vi "Measurement UI.vi"() -> ()   [LabVIEW 2022 SP3, in "Crosstalk Sweep_UI.lvlib"]
uses:
  Crosstalk Sweep_UI.lvlib
  shared/ui/controls/view.ctl
  shared/controls/digital output level units.ctl
  shared/controls/sweep profile.ctl
  UI State.ctl
  <vilib>/Utility/miscctls.llb/LVBoundsTypeDef.ctl
  <vilib>/Utility/miscctls.llb/LVPoint32TypeDef.ctl
  <vilib>/Utility/miscctls.llb/LVPointTypeDef.ctl
  shared/ui/UI Helpers.lvlib
  shared/audio popup ui/Audio Popup UI.lvlib
  shared/controls/audio controls.lvlib
panel:
  in  "view legend":T1
  out "plot point":string
  out "Sweep graph":cluster{"frequency (Hz)":dbl[], "THD+N":dbl[]}[](graph)
  out "Time domain graph":waveform(dbl)[](graph)
  out "Frequency domain graph":cluster{"f0":dbl, "df":dbl, "data":dbl[]}[](graph)
  in  "acq channel - interferrer":string="PXI1Slot4/ai0"
  in  "acq channel - victim":string="PXI1Slot4/ai1, PXI1Slot2/ai0:1"
  out "channel names":string[](array[string])
  in  "digital serial cfg file":string
  out "crosstalk (dB)":dbl[](array[numeric])
  out "frequency (Hz)":dbl[](array[numeric])
  in  "Configuration tab":enum32{"Protocol", "Measurement"}(tab)
  out "digital serial file name":string
  in  "configure digital serial":bool
  in  "master clock channel list":string caption="Master Clock Channel"
  in  "digital channel list":string caption="Digital Audio Channel"
  in  "sweep profile":T2=enum."Logarithmic" caption="Profile"
  in  "output level":dbl=-1.0 caption="Output level" format="%#_3f"
  in  "output level units":T3=enum."dBFS"
  in  "digital audio interferrer channel":i32 caption="Interferrer channel"
  in  "Interferrer channel resource":tag
  in  "Victim channel resource":tag
  in  "min settling cycles":u32 caption="Minimum settling cycles"
  in  "min settling time (s)":dbl=0.1 caption="Minimum settling time" format="%#_6ps"
  in  "number of steps":u32=20000 caption="Number of steps"
  in  "sweep start frequency (Hz)":dbl=20.0 caption="Sweep start" format="%#_6pHz"
  in  "sweep stop frequency (Hz)":dbl=20000.0 caption="Sweep stop" format="%#_6pHz"
  in  "min measurement cycles":u32 caption="Minimum measurement cycles"
  in  "acq sampling rate":dbl=51200.0 caption="Sample rate" format="%#.6pHz"
  in  "min measurement time (s)":dbl=0.1 caption="Minimum measurement time" format="%#_6ps"
  in  "lowpass filter":T4(ring) caption="Lowpass filter"
  in  "highpass filter":enum32{"DC", "AC"}(ring) caption="Highpass filter"
  in  "weighting filter":T5(ring)=enum."A-weighting" caption="Weighting filter"
  in  "load impedance":dbl=4.0 caption="Load impedance" format="%#_6p Ohms"
  in  "output range (pk-pk)":dbl=15.0 caption="Output range" format="%.3p Vpk-pk"
  out "fft - data":dbl[](array[numeric])
  out "fft - df":dbl
  out "fft - f0":dbl
  out "wfm - data":dbl[](array[numeric])
  out "wfm - dt":dbl
  out "wfm - t0":dbl
  in  "acq channel":string="PXI1Slot4/ai0"
  in  "signal phase":dbl caption="phase"
  # "hidden controls - used to sync with MeasLink"
  # "hidden indicators"
  # "Digital Serial Settings"
  # "Harware Resource"
  # "Filters"
  # "Output Sweep"
  # "Acquisition"
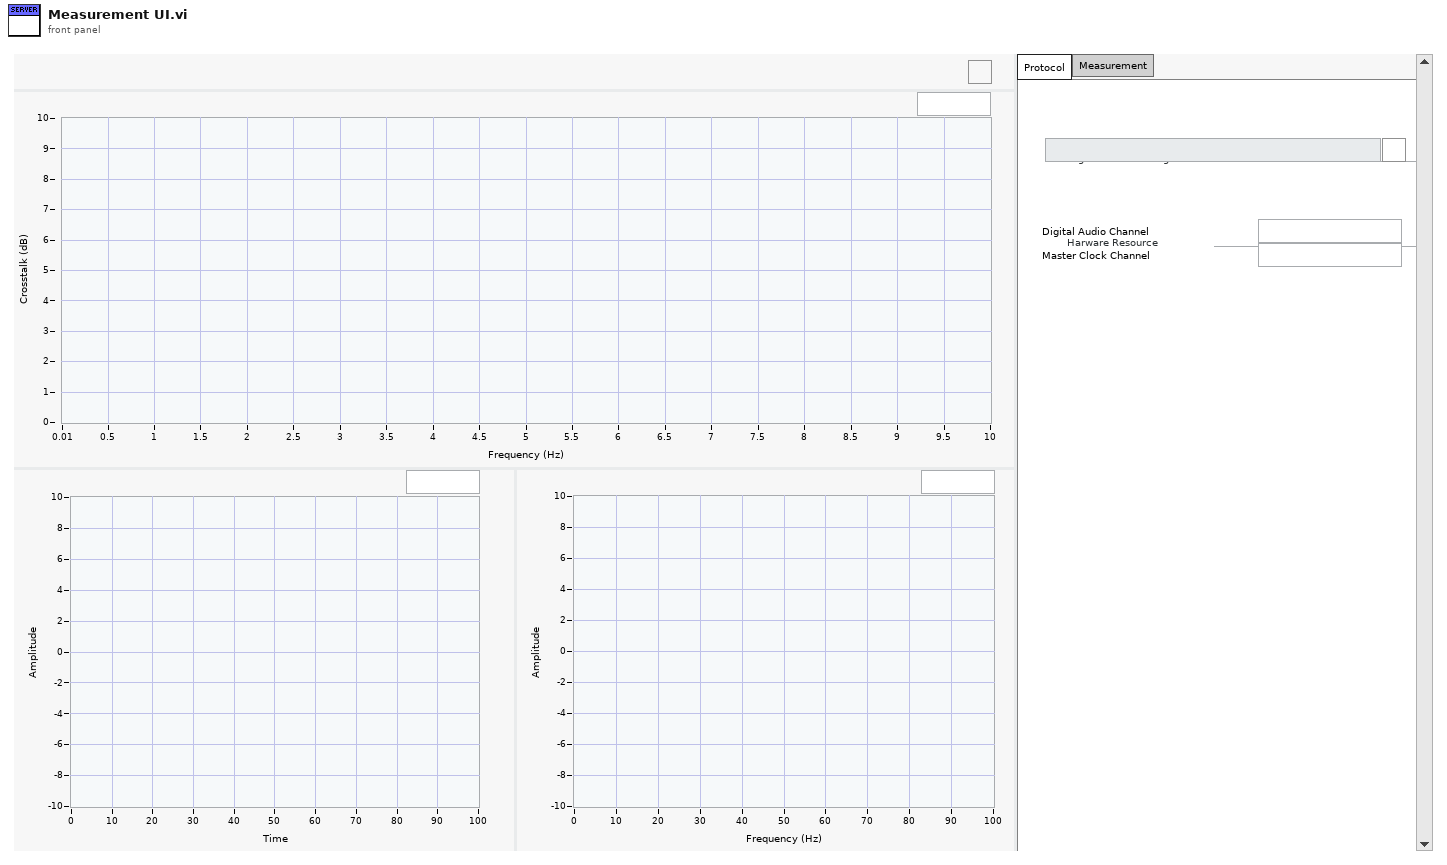
[diagram p1: front panel]
types:
  T1 = typedef "UI Helpers.lvlib/view.ctl" = bool
  T2 = typedef "audio controls.lvlib/sweep profile.ctl" = enum32{"Linear", "Logarithmic"}
  T3 = typedef "audio controls.lvlib/digital output level units.ctl" = enum32{"% FS", "dBFS", "V"}
  T4 = enum32{"No filter", "AES17 20kHz", "AES17 40kHz"}
  T5 = enum32{"Linear", "A-weighting", "B-weighting", "C-weighting"}
  T6 = typedef "Crosstalk Sweep_UI.lvlib/UI State.ctl" = cluster{"Graph Size":T7, "Legend Visible":bool, "Mouse Coords":T8, "Visible Plot Id":i32, "PostUI event occurred":bool, "digital serial cfg file":path}
  T7 = typedef "LVBoundsTypeDef.ctl" = cluster{"Width":u32, "Height":u32}
  T8 = typedef "LVPoint32TypeDef.ctl" = cluster{"Horizontal":i32, "Vertical":i32}
  T9 = typedef "LVPointTypeDef.ctl" = cluster{"Horizontal":i16, "Vertical":i16}
  T10 = typedef "Audio Popup UI.lvlib/audio settings.ctl" = cluster{"digital serial file":string}
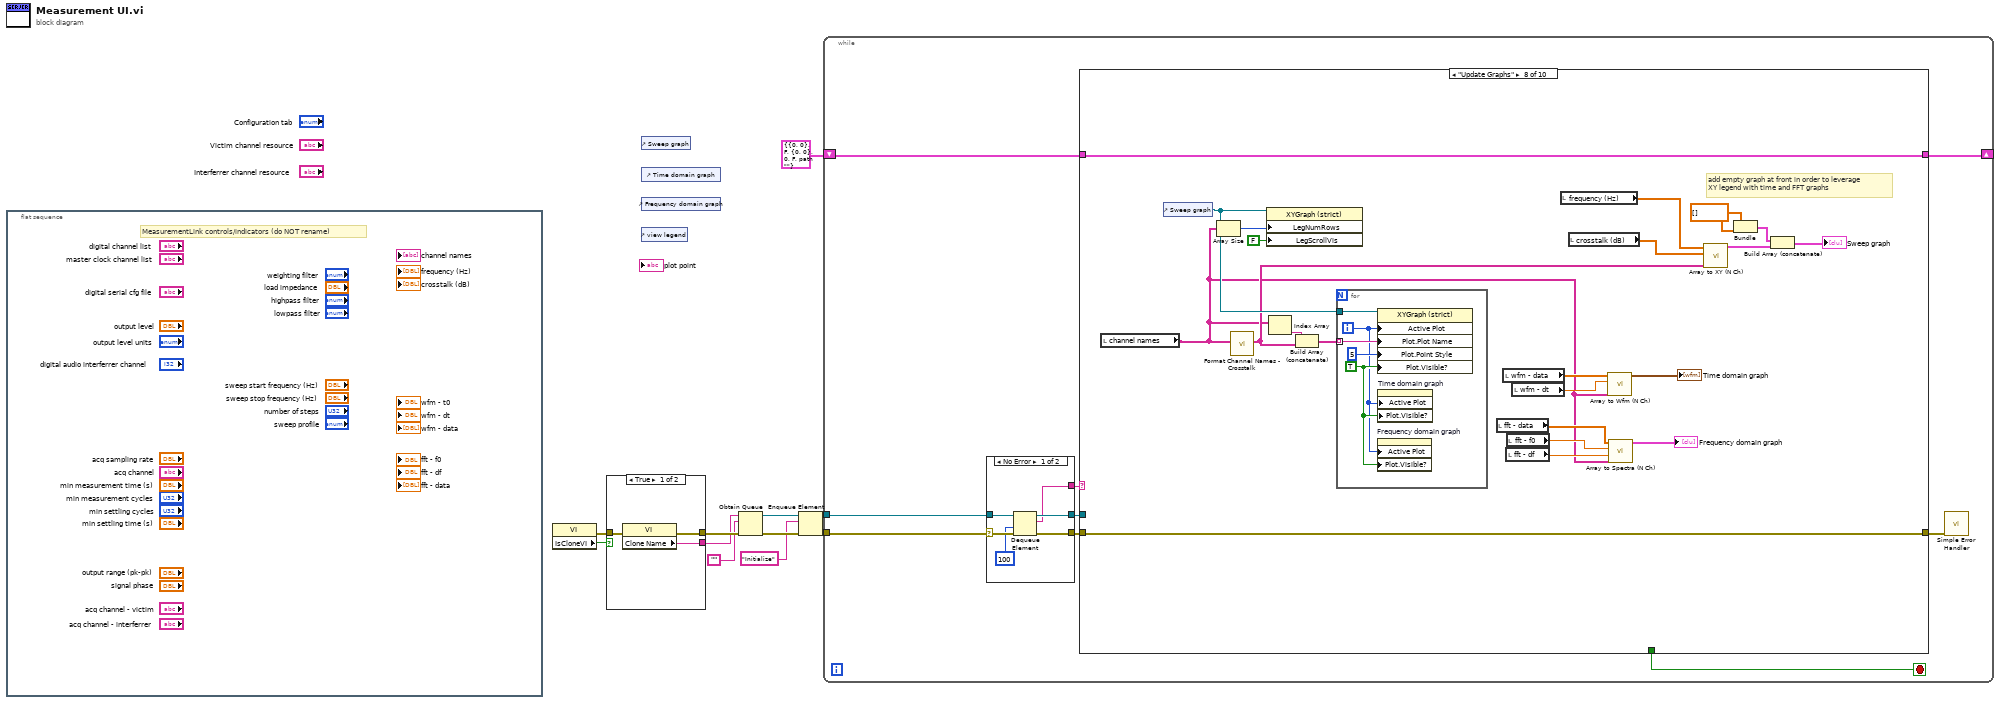
[diagram p0: block diagram]
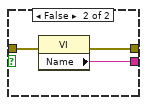
[diagram p2: hidden frame]
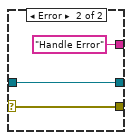
[diagram p3: hidden frame]
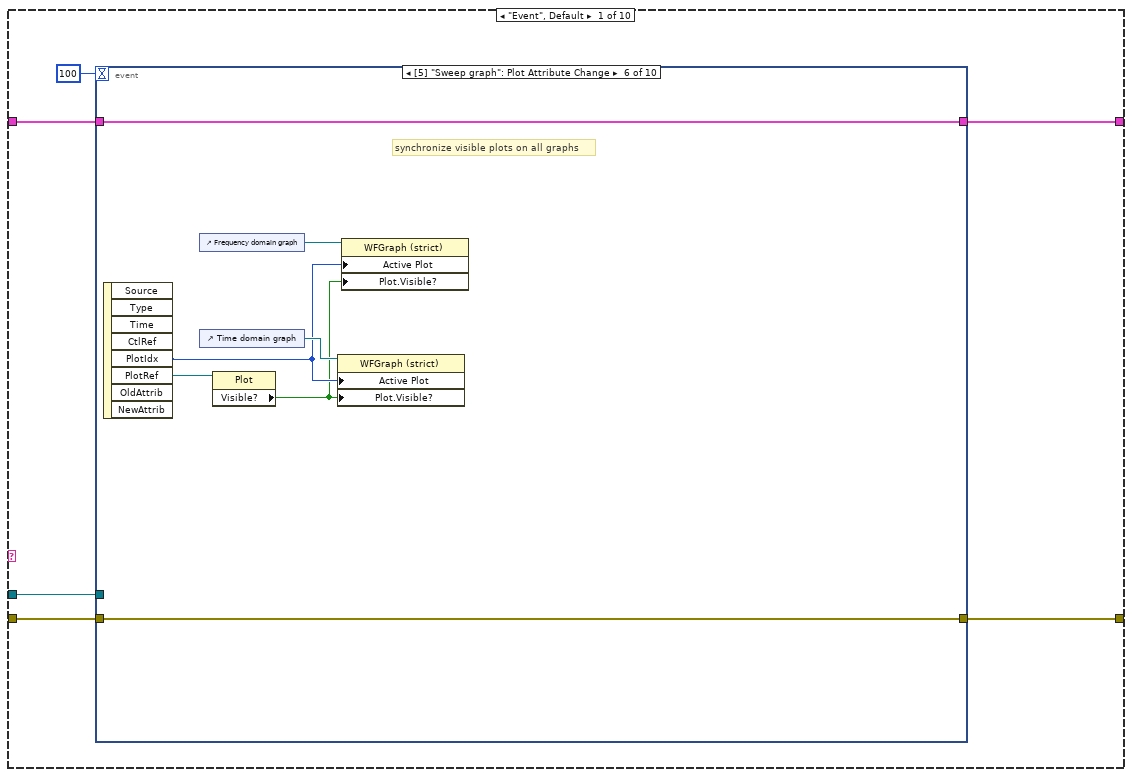
[diagram p4: hidden frame]
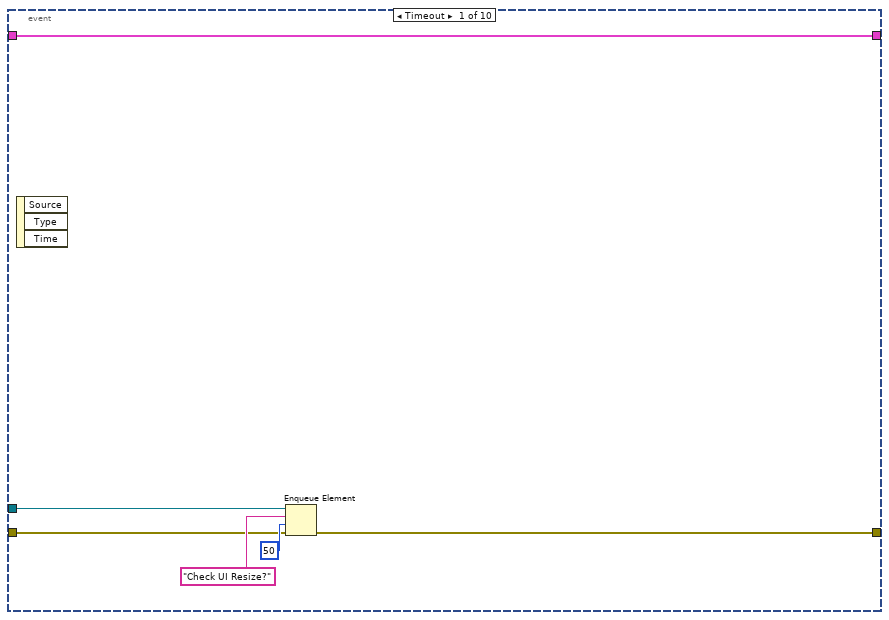
[diagram p5: hidden frame]
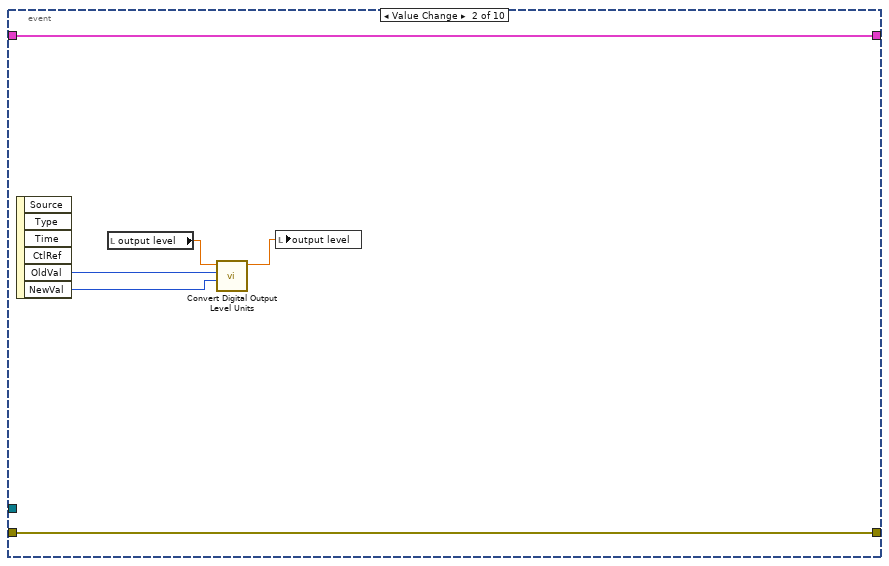
[diagram p6: hidden frame]
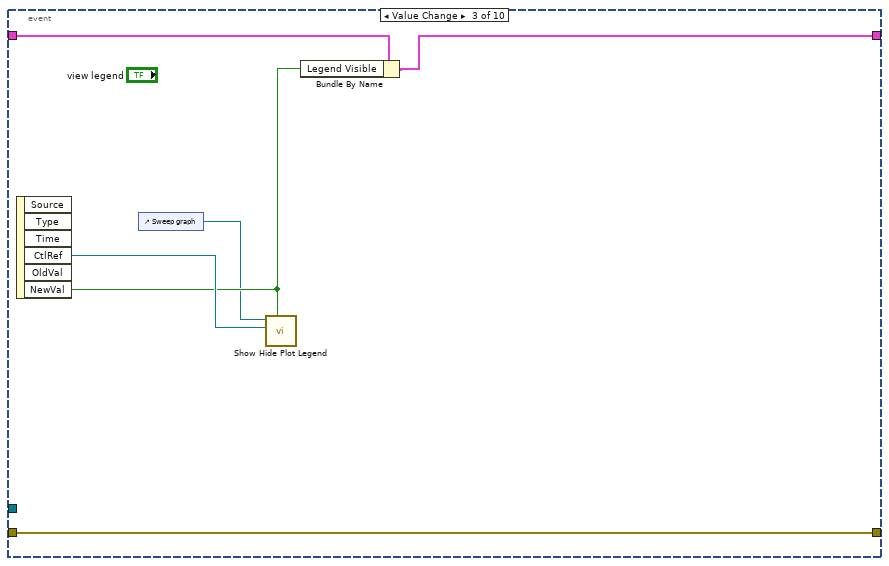
[diagram p7: hidden frame]
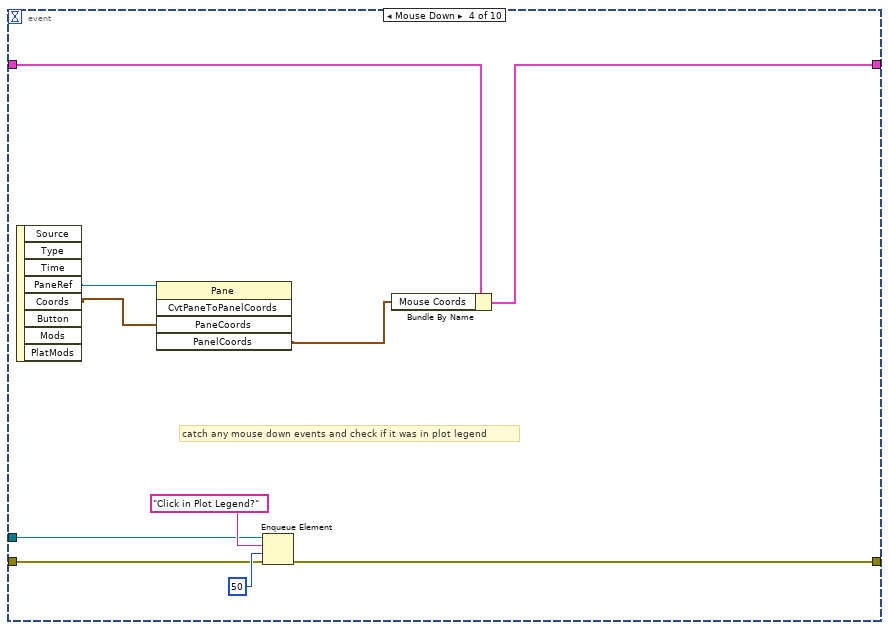
[diagram p8: hidden frame]
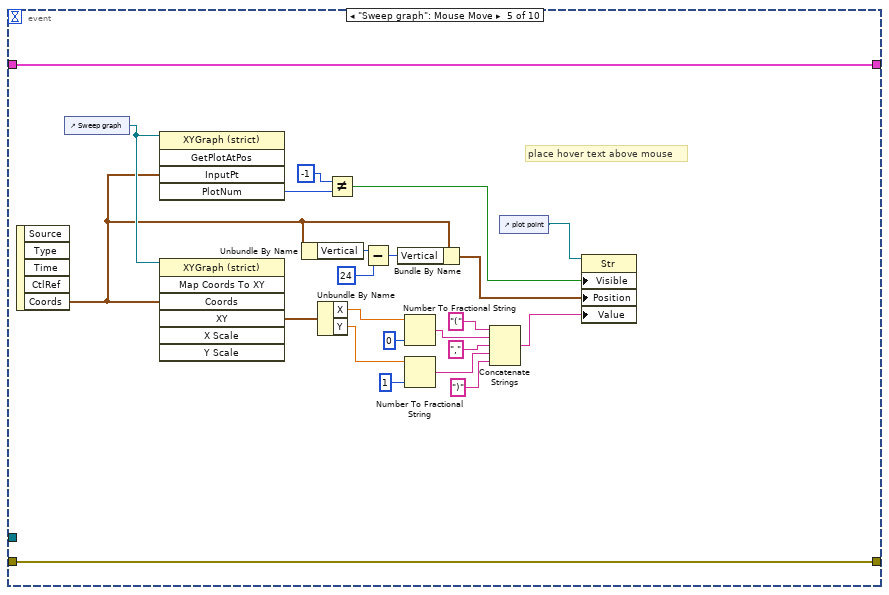
[diagram p9: hidden frame]
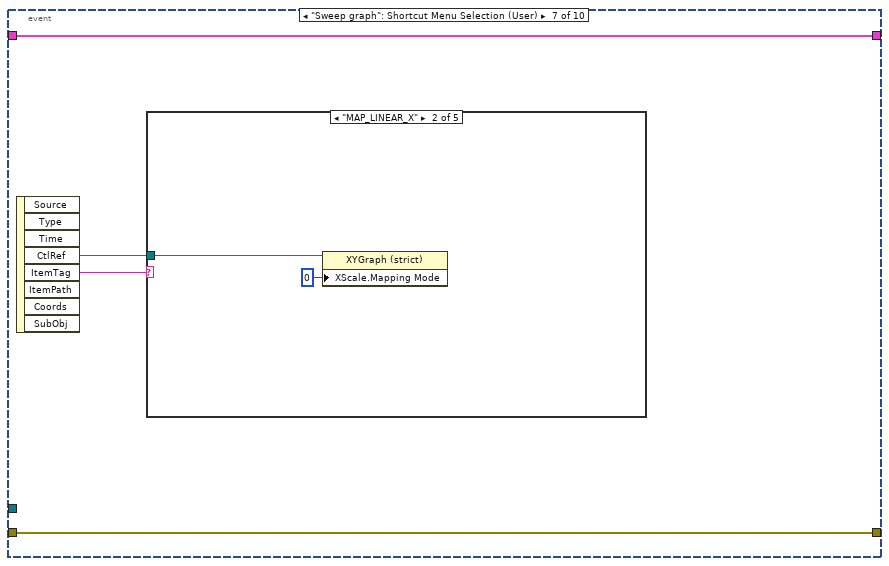
[diagram p10: hidden frame]
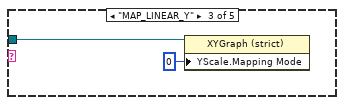
[diagram p12: hidden frame]
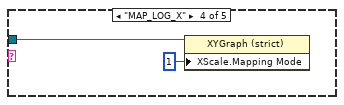
[diagram p13: hidden frame]
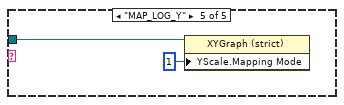
[diagram p14: hidden frame]
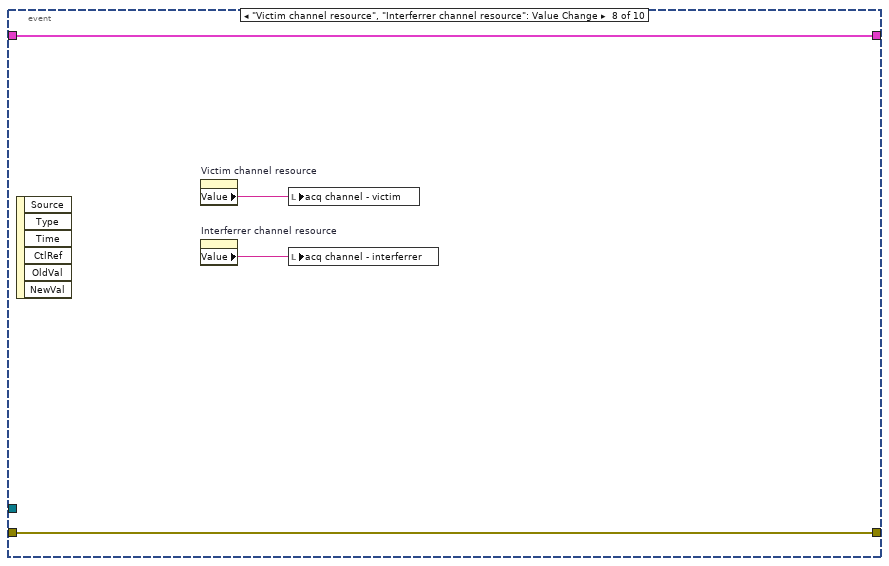
[diagram p15: hidden frame]
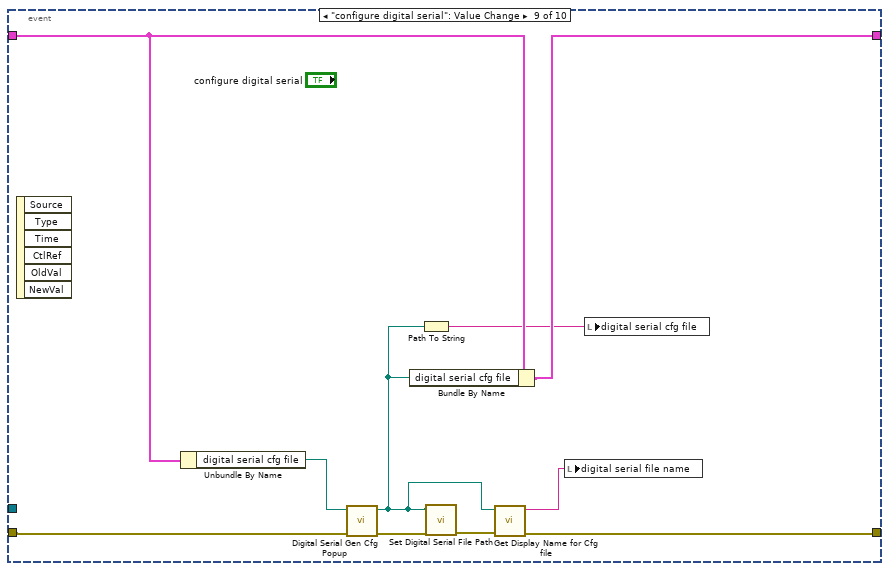
[diagram p16: hidden frame]
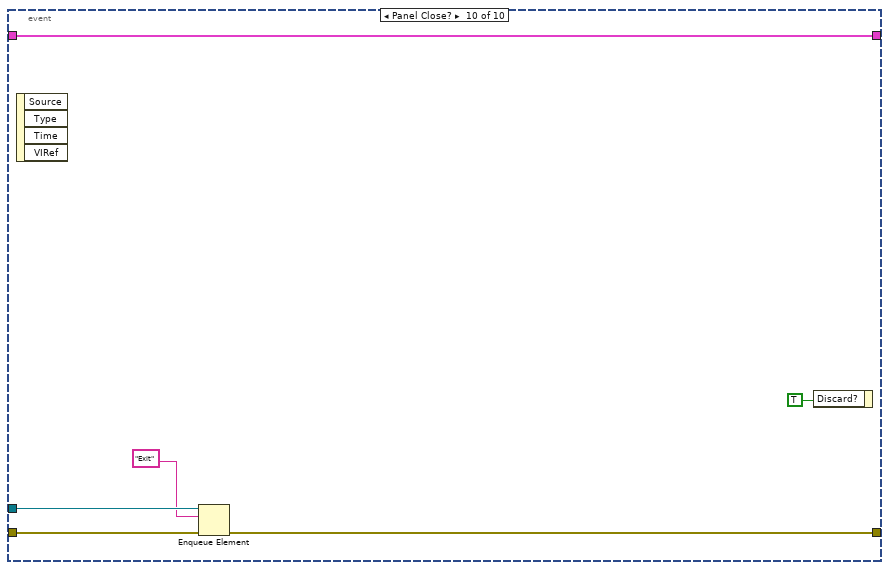
[diagram p17: hidden frame]
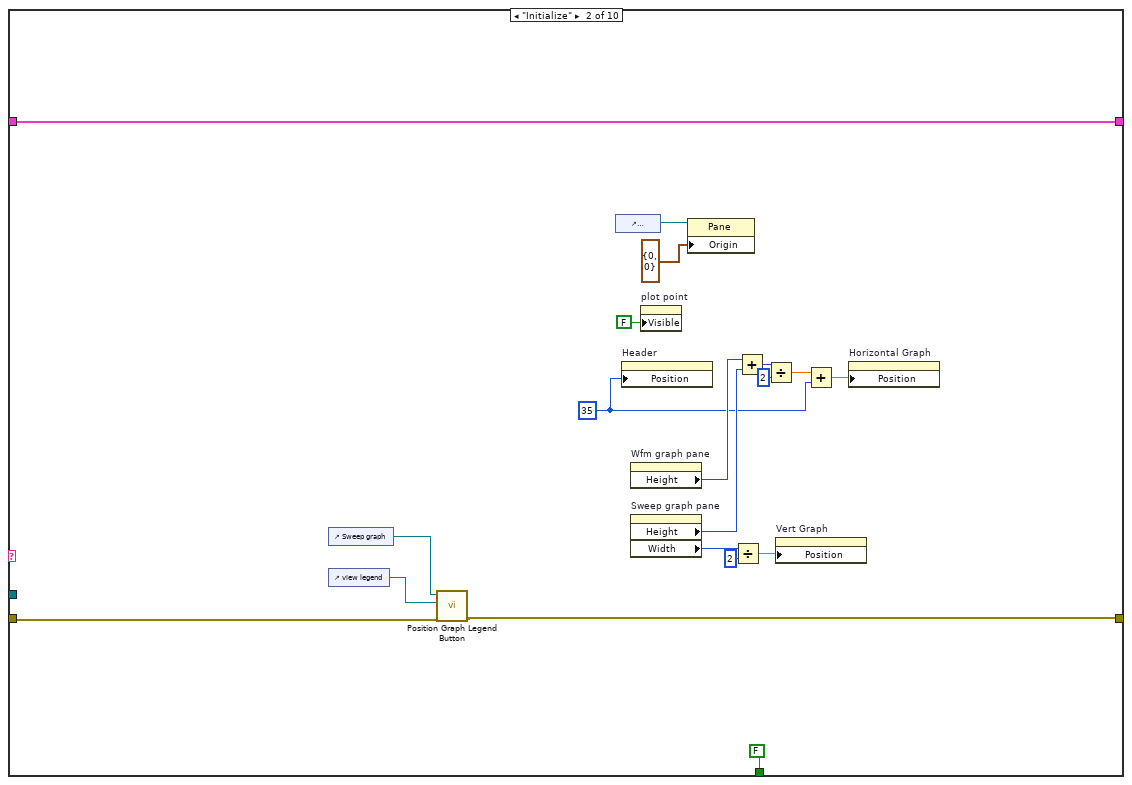
[diagram p18: hidden frame]
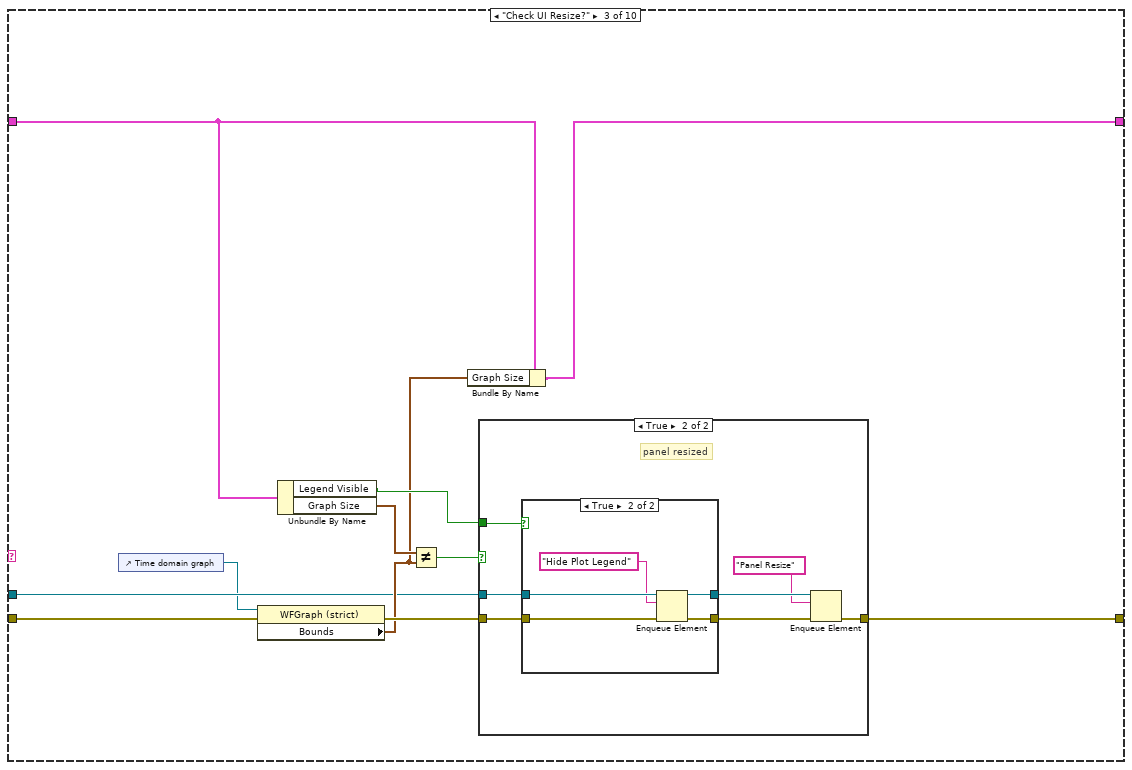
[diagram p19: hidden frame]
diagram:
  n1 = flat-sequence {
    frame #0 {
      # "MeasurementLink controls/indicators (do NOT rename)"
    }
  }
  n2 = property class="VI"() -> (error out=w2:errorcluster, "IsCloneVI"=w3:bool)  [unwired: 2 in, 1 out]
  n3 = case shown="True" w3 {
    tunnel: [w14 w17] -> w11
    tunnel: [w13 w16] -> w10
    tunnel: w2 -> [w12 w15]
    frame True {
      n4 = property class="VI"(error in=w12) -> (error out=w14:errorcluster, "Clone Name"=w13:string)  [unwired: 1 in, 1 out]
    }
    frame False {
      n5 = property class="VI"(error in=w15) -> (error out=w17:errorcluster, "Name"=w16:string)  [unwired: 1 in, 1 out]
    }
  }
  n6 = control-ref of="Sweep graph"() -> ()  [unwired: 1 out]
  n7 = control-ref of="Time domain graph"() -> ()  [unwired: 1 out]
  n8 = control-ref of="Frequency domain graph"() -> ()  [unwired: 1 out]
  n9 = control-ref of="view legend"() -> ()  [unwired: 1 out]
  n10 = Obtain Queue(name (unnamed)=w10, element data type="", error in (no error)=w11) -> (queue out=w7:refnum<queue>, error out=w9:errorcluster)  [unwired: 2 in, 1 out]
  n11 = Enqueue Element(queue=w7, element="Initialize", error in (no error)=w9) -> (queue out=w6:refnum<queue>, error out=w8:errorcluster)  [unwired: 1 in, 1 out]
  n12 = while {
    tunnel: w6 -> [w24]
    shift-right: [w20] -> _
    shift-left: T6 {"Graph Size"={"Width"=0, "Height"=0}, "Legend Visible"=FALSE, "Mouse Coords"={"Horizontal"=0, "Vertical"=0}, "Visible Plot Id"=0, "PostUI event occurred"=FALSE, "digital serial cfg file"=path ""} ("UI State") -> [w19]
    tunnel: w8 -> [w26]
    stop <- w21 stop-if-true
    n13 = case shown="No Error" w26 {
      selector: w26 -> [w32 w35]
      tunnel: [w31 w35] -> w25
      tunnel: w24 -> [w30 w34]
      tunnel: [w29 w34] -> w23
      tunnel: [w28 "Handle Error"] -> w22
      frame No Error {
        n14 = Dequeue Element(queue=w30, timeout in ms (-1)=100, error in (no error)=w32) -> (queue out=w29:refnum<queue>, element=w28:string, error out=w31:errorcluster)  [unwired: 1 out]
      }
      frame Error {
      }
    }
    n15 = case shown="\"Update Graphs\"" w22 {
      tunnel: w25 -> [w40 w133 w155 w179 w199 w207 w215 w251 w277 w279]
      tunnel: w23 -> [w38 _ w156 w180 _ _ w214 _ w275 _]
      tunnel: [w41 w132 w154 w178 w198 w204 w209 w251 w272 w279] -> w18
      tunnel: [_ FALSE _ _ _ _ _ _ TRUE _] -> w21
      tunnel: [w36 w134 w151 w177 w201 w208 w212 w264 w270 w278] -> w20
      tunnel: w19 -> [w37 w134 w152 w177 w202 w208 w213 w264 w270 w278]
      frame "Event", Default {
        n16 = event shown="[5] \"Sweep graph\": Plot Attribute Change" {
          selector: _ -> [_ _ _ _ _ _ _ _ _ _]
          dyn-events: _ -> [_ _ _ _ _ _ _ _ _ _]
          timeout: 100 -> [_ _ _ _ _ _ _ _ _ _]
          tunnel: [w44 w53 w59 w65 w92 w98 w103 w114 w116 w129] -> w41
          tunnel: w40 -> [w45 w53 w59 w67 w92 w98 w103 w114 w121 w130]
          tunnel: w38 -> [w43 _ _ w66 _ _ _ _ _ w128]
          tunnel: w37 -> [w42 w52 w56 w64 w91 w97 w102 w115 w120 w126]
          tunnel: [w42 w52 w55 w63 w91 w97 w102 w115 w119 w126] -> w36
          event Timeout {
            n17 = event-data() -> ()  [unwired: 1 in, 3 out]
            n18 = Enqueue Element(queue=w43, element="Check UI Resize?", timeout in ms (-1)=50, error in (no error)=w45) -> (error out=w44:errorcluster)  [unwired: 2 out]
          }
          event Value Change {
            n19 = event-data() -> ("OldVal"=w50:T3, "NewVal"=w49:T3)  [unwired: 1 in, 4 out]
            n20 = local read "output level"() -> (w51:dbl)
            n21 = call "Convert Digital Output Level Units.vi"("new output level units"=w49, "previous output level units"=w50, "previous output level"=w51) -> ("new output level"=w48:dbl)  [unwired: 8 in]
            n22 = local write "output level"(w48) -> ()
          }
          event Value Change {
            n23 = event-data() -> ("CtlRef"=w58:refnum<vi>, "NewVal"=w57:T1)  [unwired: 1 in, 4 out]
            n24 = control-ref of="Sweep graph"() -> (w54:refnum<vi>)
            n25 = call "Show Hide Plot Legend.vi"("show"=w57, "view reference"=w58, "graph reference"=w54) -> ()  [unwired: 8 in, 1 out]
            n26 = Bundle By Name(cluster=w56, "Legend Visible"=w57) -> (w55:T6)
          }
          event Mouse Down {
            # "catch any mouse down events and check if it was in plot legend"
            n27 = event-data() -> ("PaneRef"=w62:refnum<vi>, "Coords"=w61:T8)  [unwired: 1 in, 6 out]
            n28 = invoke class="Pane" method="CvtPaneToPanelCoords"(reference=w62, "PaneCoords"=w61) -> ("PanelCoords"=w60:T9)  [unwired: 3 in, 4 out]
            n29 = Enqueue Element(queue=w66, element="Click in Plot Legend?", timeout in ms (-1)=50, error in (no error)=w67) -> (error out=w65:errorcluster)  [unwired: 2 out]
            n30 = Bundle By Name(cluster=w64, "Mouse Coords"=w60) -> (w63:T6)
          }
          event "Sweep graph": Mouse Move {
            # "place hover text above mouse"
            n31 = event-data() -> ("Coords"=w71:T8)  [unwired: 1 in, 4 out]
            n32 = control-ref of="Sweep graph"() -> (w72:refnum<vi>)
            n33 = invoke class="XYGraph (strict)" method="GetPlotAtPos"(reference=w72, "InputPt"=w71) -> ("PlotNum"=w89:i32)  [unwired: 3 in, 4 out]
            n34 = invoke class="XYGraph (strict)" method="Map Coords To XY"(reference=w72, "Coords"=w71) -> ("XY"=w90:cluster{"X":dbl, "Y":dbl})  [unwired: 5 in, 6 out]
            n35 = Unbundle By Name(w71) -> ("Vertical"=w76:i32)
            n36 = Unbundle By Name(w90) -> ("X"=w79:dbl, "Y"=w78:dbl)
            n37 = Not Equal?(x=-1, y=w89) -> (x != y?=w87:bool)
            n38 = Subtract(x=w76, y=24) -> (x-y=w75:i32)
            n39 = Bundle By Name(cluster=w71, "Vertical"=w75) -> (w77:T8)
            n40 = Number To Fractional String(number=w79, precision (6)=i16 0) -> (F-format string=w85:string)  [unwired: 2 in]
            n41 = Number To Fractional String(number=w78, precision (6)=i16 1) -> (F-format string=w83:string)  [unwired: 2 in]
            n42 = Concatenate Strings("(" ("string"), w85, "," ("string"), w83, ")" ("string")) -> (w80:string)
            n43 = control-ref of="plot point"() -> (w73:refnum<vi>)
            n44 = property on="Property Node" class="Str"(reference=w73, "Visible"=w87, "Position"=w77, "Value"=w80) -> ()  [unwired: 1 in, 2 out]
          }
          event "Sweep graph": Plot Attribute Change {
            # "synchronize visible plots on all graphs"
            n45 = event-data() -> ("PlotIdx"=w94:i32, "PlotRef"=w99:refnum<vi>)  [unwired: 1 in, 6 out]
            n46 = control-ref of="Frequency domain graph"() -> (w95:refnum<vi>)
            n47 = control-ref of="Time domain graph"() -> (w96:refnum<vi>)
            n48 = property class="Plot"(reference=w99) -> ("Visible?"=w93:bool)  [unwired: 1 in, 2 out]
            n49 = property on="Property Node" class="WFGraph (strict)"(reference=w96, "Active Plot"=w94, "Plot.Visible?"=w93) -> ()  [unwired: 1 in, 2 out]
            n50 = property on="Property Node" class="WFGraph (strict)"(reference=w95, "Active Plot"=w94, "Plot.Visible?"=w93) -> ()  [unwired: 1 in, 2 out]
          }
          event "Sweep graph": Shortcut Menu Selection (User) {
            n51 = event-data() -> ("CtlRef"=w100:refnum<vi>, "ItemTag"=w101:string)  [unwired: 1 in, 6 out]
            n52 = case shown="\"MAP_LINEAR_X\"" w101 {
              tunnel: w100 -> [_ w105 w107 w109 w111]
              frame "", Default {
              }
              frame "MAP_LINEAR_X" {
                n53 = property class="XYGraph (strict)"(reference=w105, "XScale.Mapping Mode"=u8 0 ("X Scale.Mapping Mode")) -> ()  [unwired: 1 in, 2 out]
              }
              frame "MAP_LINEAR_Y" {
                n54 = property class="XYGraph (strict)"(reference=w107, "YScale.Mapping Mode"=u8 0 ("X Scale.Mapping Mode")) -> ()  [unwired: 1 in, 2 out]
              }
              frame "MAP_LOG_X" {
                n55 = property class="XYGraph (strict)"(reference=w109, "XScale.Mapping Mode"=u8 1 ("X Scale.Mapping Mode")) -> ()  [unwired: 1 in, 2 out]
              }
              frame "MAP_LOG_Y" {
                n56 = property class="XYGraph (strict)"(reference=w111, "YScale.Mapping Mode"=u8 1 ("X Scale.Mapping Mode")) -> ()  [unwired: 1 in, 2 out]
              }
            }
          }
          event "Victim channel resource", "Interferrer channel resource": Value Change {
            n57 = event-data() -> ()  [unwired: 1 in, 6 out]
            n58 = property on="Victim channel resource" class="DAQmxName"() -> ("Value"=w112:string)  [unwired: 2 in, 2 out]
            n59 = property on="Interferrer channel resource" class="DAQmxName"() -> ("Value"=w113:string)  [unwired: 2 in, 2 out]
            n60 = local write "acq channel - victim"(w112) -> ()
            n61 = local write "acq channel - interferrer"(w113) -> ()
          }
          event "configure digital serial": Value Change {
            n62 = event-data() -> ()  [unwired: 1 in, 6 out]
            n63 = Unbundle By Name(w120) -> ("digital serial cfg file"=w125:path)
            n64 = call "Digital Serial Gen Cfg Popup.vi"("error in (no error)"=w121, "config file in"=w125) -> ("error out"=w124:errorcluster, "config file out"=w122:path)  [unwired: 7 in, 1 out]
            n65 = Bundle By Name(cluster=w120, "digital serial cfg file"=w122) -> (w119:T6)
            n66 = Path To String(path=w122) -> (string=w118:string)
            n67 = call "Set Digital Serial File Path.vi"("error in (no error)"=w124, "digital serial file"=w122) -> ("error out"=w123:errorcluster)  [unwired: 9 in]
            n68 = call "Get Display Name for Cfg file.vi"("error in (no error)"=w123, "file path"=w122) -> ("error out"=w116:errorcluster, "display string"=w117:string)  [unwired: 8 in]
            n69 = local write "digital serial file name"(w117) -> ()
            n70 = local write "digital serial cfg file"(w118) -> ()
          }
          event Panel Close? {
            n71 = event-data() -> ()  [unwired: 1 in, 4 out]
            n72 = Enqueue Element(queue=w128, element="Exit", error in (no error)=w130) -> (error out=w129:errorcluster)  [unwired: 1 in, 2 out]
            n73 = event-data("Discard?"=TRUE) -> ()  [unwired: 1 in, 1 out]
          }
        }
      }
      frame "Initialize" {
        w138 = 35 ("Splitter Position")
        n74 = control-ref of="Sweep graph"() -> (w139:refnum<vi>)
        n75 = control-ref of="view legend"() -> (w149:refnum<vi>)
        n76 = call "Position Graph Legend Button.vi"("error in (no error)"=w133, "view legend"=w149, "graph"=w139) -> ("error out"=w132:errorcluster)  [unwired: 8 in]
        n77 = control-ref of="Configuration Pane"() -> (w137:refnum<vi>)
        n78 = property on="Header" class="Splitter"("Position"=w138) -> ()  [unwired: 2 in, 2 out]
        n79 = property on="Wfm graph pane" class="Pane"() -> ("Height"=w142:u32)  [unwired: 2 in, 2 out]
        n80 = property on="Sweep graph pane" class="Pane"() -> ("Height"=w141:u32, "Width"=w144:u32)  [unwired: 2 in, 2 out]
        n81 = property on="plot point" class="Str"("Visible"=FALSE) -> ()  [unwired: 2 in, 2 out]
        n82 = property class="Pane"(reference=w137, "Origin"=T9 {"Horizontal"=0, "Vertical"=0}) -> ()  [unwired: 1 in, 2 out]
        n83 = Divide(x=w144, y=2) -> (x/y=w143:dbl)
        n84 = Add(x=w142, y=w141) -> (x+y=w140:u32)
        n85 = Divide(x=w140, y=2) -> (x/y=w147:dbl)
        n86 = property on="Vert Graph" class="Splitter"("Position"=w143) -> ()  [unwired: 2 in, 2 out]
        n87 = Add(x=w147, y=w138) -> (x+y=w146:dbl)
        n88 = property on="Horizontal Graph" class="Splitter"("Position"=w146) -> ()  [unwired: 2 in, 2 out]
      }
      frame "Check UI Resize?" {
        n89 = control-ref of="Time domain graph"() -> (w153:refnum<vi>)
        n90 = property on="Property Node" class="WFGraph (strict)"(reference=w153, error in=w155) -> (error out=w161:errorcluster, "Bounds"=w157:T7)  [unwired: 1 out]
        n91 = Unbundle By Name(w152) -> ("Legend Visible"=w159:bool, "Graph Size"=w158:T7)
        n92 = Not Equal?(x=w158, y=w157) -> (x != y?=w160:bool)
        n93 = Bundle By Name(cluster=w152, "Graph Size"=w157) -> (w151:T6)
        n94 = case shown="True" w160 {
          tunnel: w161 -> [w162 w169]
          tunnel: [w162 w164] -> w154
          tunnel: w159 -> [_ w167]
          tunnel: w156 -> [_ w168]
          frame False {
            # "no resize"
          }
          frame True {
            # "panel resized"
            n95 = case shown="True" w167 {
              tunnel: w169 -> [w171 w176]
              tunnel: [w171 w175] -> w166
              tunnel: w168 -> [w170 w174]
              tunnel: [w170 w172] -> w165
              frame False {
              }
              frame True {
                n96 = Enqueue Element(queue=w174, element="Hide Plot Legend", error in (no error)=w176) -> (queue out=w172:refnum<queue>, error out=w175:errorcluster)  [unwired: 1 in, 1 out]
              }
            }
            n97 = Enqueue Element(queue=w165, element="Panel Resize", error in (no error)=w166) -> (error out=w164:errorcluster)  [unwired: 1 in, 2 out]
          }
        }
      }
      frame "Click in Plot Legend?" {
        n98 = Unbundle By Name(w177) -> ("Legend Visible"=w181:bool, "Mouse Coords"=w182:T8)
        n99 = case shown="True" w181 {
          tunnel: w182 -> [_ w189]
          tunnel: w180 -> [_ w186]
          tunnel: w179 -> [w183 w190]
          tunnel: [w183 w185] -> w178
          frame False {
            # "legend not visible; do nothing"
          }
          frame True {
            # "check if mouse down in legend"
            n100 = control-ref of="Sweep graph"() -> (w184:refnum<vi>)
            n101 = call "Check if Click in Graph Legend.vi"("error in (no error)"=w190, "Mouse Coords"=w189, "WaveformGraph"=w184) -> ("error out"=w187:errorcluster, "click in legend?"=w188:bool)  [unwired: 7 in]
            n102 = case shown="True" w188 {
              tunnel: w187 -> [w194 w195]
              tunnel: w186 -> [w193 _]
              tunnel: [w192 w195] -> w185
              frame False {
                n103 = Enqueue Element(queue=w193, element="Hide Plot Legend", error in (no error)=w194) -> (error out=w192:errorcluster)  [unwired: 1 in, 2 out]
              }
              frame True {
                # "inside legend; do nothing"
              }
            }
          }
        }
      }
      frame "Hide Plot Legend" {
        n104 = control-ref of="Sweep graph"() -> (w196:refnum<vi>)
        n105 = control-ref of="view legend"() -> (w197:refnum<vi>)
        n106 = call "Show Hide Plot Legend.vi"("show"=FALSE, "error in (no error)"=w199, "view reference"=w197, "graph reference"=w196) -> ("error out"=w198:errorcluster)  [unwired: 7 in]
        n107 = Bundle By Name(cluster=w202, "Legend Visible"=FALSE ("legend visible")) -> (w201:T6)
      }
      frame "Panel Resize" {
        n108 = control-ref of="Sweep graph"() -> (w206:refnum<vi>)
        n109 = control-ref of="view legend"() -> (w205:refnum<vi>)
        n110 = call "Position Graph Legend Button.vi"("error in (no error)"=w207, "view legend"=w205, "graph"=w206) -> ("error out"=w204:errorcluster)  [unwired: 8 in]
      }
      frame "Post UI Update" {
        # "This case will be triggered, after framework updates the User interface with result values."
        n111 = for {
          tunnel: w214 -> [w240]
          shift-right: [w239] -> w210
          shift-left: w215 -> [w241]
          tunnel: string[] ["Update Graphs"] -> [w238] mode=indexing
          n112 = Enqueue Element(queue=w240, element=w238, timeout in ms (-1)=50, error in (no error)=w241) -> (error out=w239:errorcluster)  [unwired: 2 out]
        }
        n113 = Unbundle By Name(w213) -> ("PostUI event occurred"=w211:bool)
        n114 = case shown="False" w211 {
          tunnel: w213 -> [w229 w237]
          tunnel: [w228 w237] -> w212
          tunnel: w210 -> [w225 w236]
          tunnel: [w220 w236] -> w209
          frame False {
            # "Initialize the DAQmx channel control"
            # "do this on first PostUI Event (happens when panel loads)"
            n115 = local read "digital serial cfg file"() -> (w222:string)
            n116 = local read "acq channel - victim"() -> (w218:string)
            n117 = local read "acq channel - interferrer"() -> (w217:string)
            n118 = Empty String/Path?(string/path=w222) -> (empty?=w221:bool)
            n119 = case shown="True" w221 {
              tunnel: w225 -> [w231 w235]
              tunnel: [w231 w233] -> w226
              tunnel: w222 -> [w230 _]
              tunnel: [w230 w232] -> w223
              frame False {
              }
              frame True {
                n120 = call "Get Audio Settings.vi"("error in (no error)"=w235) -> ("error out"=w233:errorcluster, "audio settings"=w234:T10)  [unwired: 9 in]
                n121 = Unbundle By Name(w234) -> ("digital serial file"=w232:string)
              }
            }
            n122 = property on="Interferrer channel resource" class="DAQmxName"("Value"=w217) -> ()  [unwired: 2 in, 2 out]
            n123 = property on="Victim channel resource" class="DAQmxName"("Value"=w218) -> ()  [unwired: 2 in, 2 out]
            n124 = String To Path(string=w223) -> (path=w224:path)
            n125 = local write "digital serial cfg file"(w223) -> ()
            n126 = call "Get Display Name for Cfg file.vi"("error in (no error)"=w226, "file path"=w224) -> ("error out"=w220:errorcluster, "display string"=→"digital serial file name":string)  [unwired: 8 in]
            n127 = Bundle By Name(cluster=w229, "PostUI event occurred"=TRUE, "digital serial cfg file"=w224) -> (w228:T6)
          }
          frame True {
          }
        }
      }
      frame "Update Graphs" {
        w243 = dbl[] []
        # "add empty graph at front in order to leverage \nXY legend with time and FFT graphs"
        n128 = local read "channel names"() -> (w248:string[])
        n129 = control-ref of="Sweep graph"() -> (w263:refnum<vi>)
        n130 = Array Size(array=w248) -> (size(s)=w262:i32)
        n131 = call "Format Channel Names - Crosstalk.vi"("names in"=w248) -> ("names out"=w249:string[])  [unwired: 10 in]
        n132 = property class="XYGraph (strict)"(reference=w263, "LegNumRows"=w262, "LegScrollVis"=FALSE ("Legend:Scrollbar Visible")) -> ()  [unwired: 1 in, 2 out]
        n133 = Index Array(array=w248) -> (element=w247:string)  [unwired: 1 in]
        n134 = Build Array (concatenate)(w247, w249) -> (w250:string[])
        n135 = for {
          tunnel: w250 -> [w269] mode=indexing
          tunnel: w263 -> [w268]
          i -> [w265]
          w266 = TRUE ("Plot.Visible")
          n136 = property on="Property Node" class="XYGraph (strict)"(reference=w268, "Active Plot"=w265, "Plot.Plot Name"=w269, "Plot.Point Style"=u8 5, "Plot.Visible?"=w266) -> ()  [unwired: 1 in, 2 out]
          n137 = property on="Frequency domain graph" class="WFGraph (strict)"("Active Plot"=w265, "Plot.Visible?"=w266) -> ()  [unwired: 2 in, 2 out]
          n138 = property on="Time domain graph" class="WFGraph (strict)"("Active Plot"=w265, "Plot.Visible?"=w266) -> ()  [unwired: 2 in, 2 out]
        }
        n139 = local read "fft - data"() -> (w253:dbl[])
        n140 = local read "wfm - data"() -> (w258:dbl[])
        n141 = local read "fft - df"() -> (w255:dbl)
        n142 = local read "fft - f0"() -> (w254:dbl)
        n143 = local read "wfm - dt"() -> (w257:dbl)
        n144 = local read "frequency (Hz)"() -> (w260:dbl[])
        n145 = local read "crosstalk (dB)"() -> (w259:dbl[])
        n146 = call "Array to Wfm (N Ch).vi"("channel names"=w248, "dt"=w257, "array"=w258) -> ("waveforms"=→"Time domain graph":waveform(dbl)[])  [unwired: 8 in]
        n147 = call "Array to Spectra (N Ch).vi"("channel names"=w248, "df"=w255, "f0"=w254, "data"=w253) -> ("spectra"=→"Frequency domain graph":cluster{"f0":dbl, "df":dbl, "data":dbl[]}[])  [unwired: 7 in]
        n148 = call "Array to XY (N Ch).vi"("channel names"=w249, "Y data"=w259, "X data"=w260) -> ("XY plots"=w246:cluster{"X data":dbl[], "Y data":dbl[]}[])  [unwired: 8 in]
        n149 = Bundle(w243, w243) -> (w244:cluster{dbl[], dbl[]})  [unwired: 1 in]
        n150 = Build Array (concatenate)(w244, w246) -> (→"Sweep graph":cluster{"X data":dbl[], "Y data":dbl[]}[])
      }
      frame "Exit" {
        # "This case is triggered to close the User Interface from framework"
        n151 = Flush Queue(queue=w275, error in (no error)=w277) -> (queue out=w274:refnum<queue>, error out=w273:errorcluster)  [unwired: 1 out]
        n152 = Release Queue(queue=w274, force destroy? (F)=TRUE, error in (no error)=w273) -> (error out=w272:errorcluster)  [unwired: 2 out]
      }
      frame "Handle Error" {
      }
    }
    n153 = call <vilib>:"Simple Error Handler.vi"("error in (no error)"=w18) -> ()  [unwired: 4 in, 5 out]
  }
